vi "Read Parameter Filter.vi"(8 "error in (no error)":errorcluster, 11 "Camera Actor in":refnum<class "Camera Actor.lvclass">) -> (0 "error out":errorcluster, 2 "Parameter Filter":T1, 3 "Camera Actor out":refnum<class "Camera Actor.lvclass">)   [LabVIEW 2014, in "Camera Actor.lvlib" / "Camera Actor.lvclass"]
uses:
  Camera Actor.lvclass
  Parameter Filters.ctl
  Camera Actor.lvclass/Camera Actor.ctl
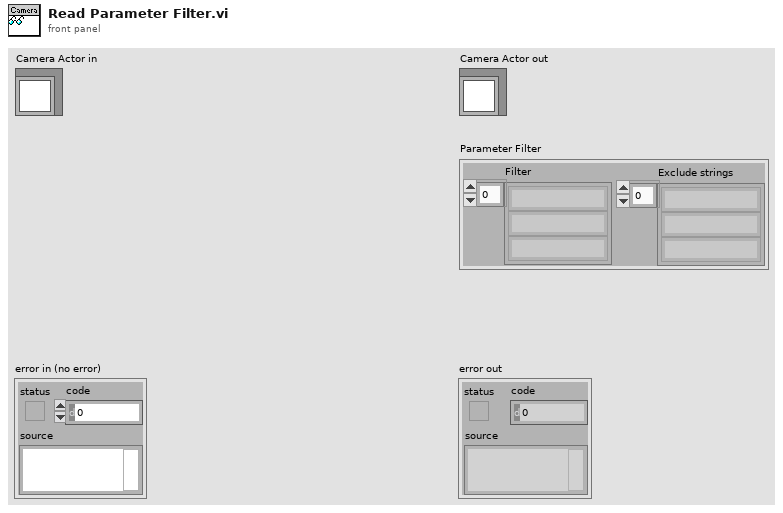
[diagram p1: front panel]
types:
  T1 = typedef "Camera Actor.lvlib/Camera Actor.lvclass/Parameter Filters.ctl" = cluster{"Filter":string[], "Exclude strings":string[]}
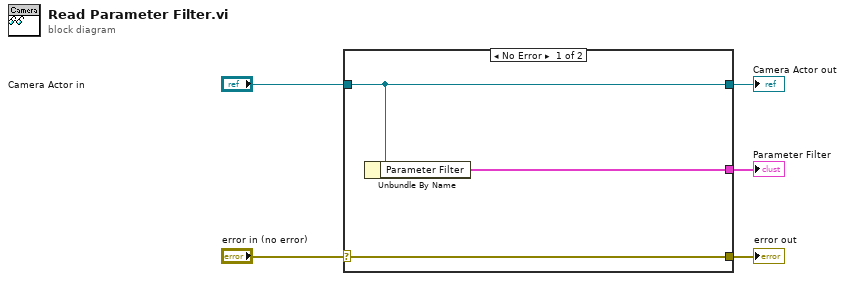
[diagram p0: block diagram]
diagram:
  n1 = case shown="No Error" "error in (no error)" {
    selector: "error in (no error)" -> [w8 w9]
    tunnel: [w8 w9] -> w4
    tunnel: [w7 w10] -> w2
    tunnel: "Camera Actor in" -> [w7 w10]
    tunnel: [w6 _] -> w1
    frame No Error {
      n2 = Unbundle By Name(w7) -> ("Parameter Filter"=w6:T1)
    }
    frame Error {
    }
  }
  "error out" <- w4
  "Camera Actor out" <- w2
  "Parameter Filter" <- w1
